vi "Start Run in DAQ.vi"(6 "Total timeout":i32, 8 "error in (no error)":errorcluster, 11 "DAQ Control in":refnum<class "DAQ Control.lvclass">) -> (0 "error out":errorcluster, 1 "TCP Port Number":u32, 2 "Run Number":u32, 3 "DAQ Control out":refnum<class "DAQ Control.lvclass">, 4 "Data storage path":string, 5 "Run Active?":bool)   [LabVIEW 2026, in "TALOS.lvlib" / "Interfaces.lvlib" / "DAQ Control.lvclass"]
uses:
  DAQ Control.lvclass
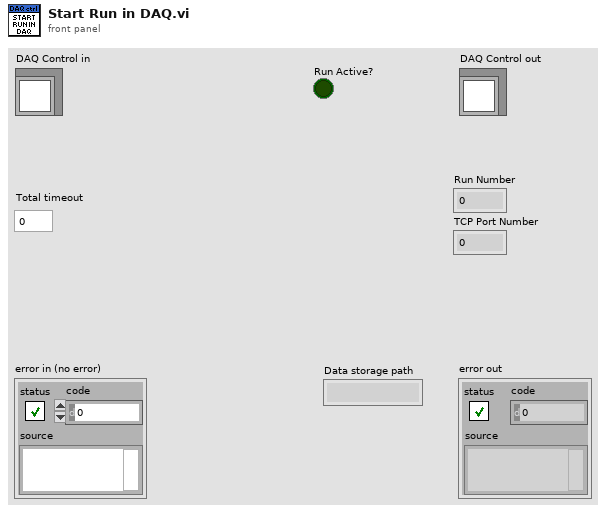
[diagram p1: front panel]
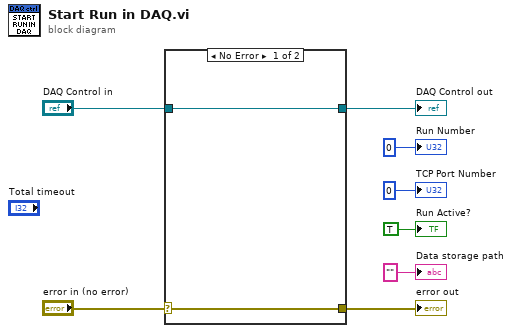
[diagram p0: block diagram]
diagram:
  n1 = case shown="No Error" "error in (no error)" {
    selector: "error in (no error)" -> [w9 w12]
    tunnel: [w9 w12] -> w7
    tunnel: [w10 w11] -> w5
    tunnel: "DAQ Control in" -> [w10 w11]
    frame No Error {
    }
    frame Error {
    }
  }
  "error out" <- w7
  "DAQ Control out" <- w5
  "Run Number" <- u32 0 ("Run Number")
  "TCP Port Number" <- u32 0 ("TCP Port Number")
  "Data storage path" <- "" ("Data storage path")
  "Run Active?" <- TRUE
